vi "dispose context.vi"(8 "error in":errorcluster, 11 "engine context out":refnum<class "engine context.lvclass">) -> (0 "error out":errorcluster)   [LabVIEW 2016, in "engine context.lvclass"]
uses:
  engine context.lvclass
  engine context.lvclass/engine context.ctl
  dllwrapper/library path.vi
  <vilib>/Utility/error.llb/Error Cluster From Error Code.vi
  dllwrapper/async tls dl.lvlib
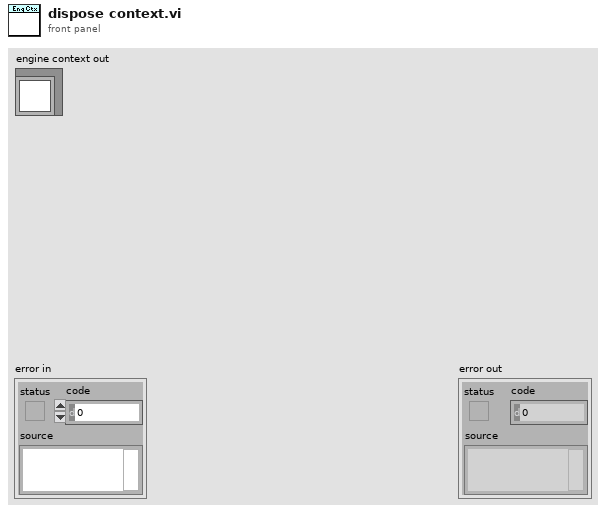
[diagram p1: front panel]
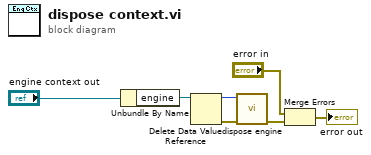
[diagram p0: block diagram]
diagram:
  n1 = Unbundle By Name("engine context out") -> ("engine"=w6:refnum<data-value>)
  n2 = Delete Data Value Reference(data value reference=w6) -> (data value=w5:u64, error out=w4:errorcluster)  [unwired: 1 in]
  n3 = call "dispose engine.vi"("error in"=w4, "engine"=w5) -> ("error out"=w3:errorcluster)  [unwired: 9 in]
  n4 = Merge Errors("error in", w3) -> (→"error out":errorcluster)
